vi "Max and Min (multiple).vi"(8 "error in (no error)":errorcluster, 11 "XY-data":cluster{"X-array":dbl[], "Y-array":dbl[]}[](array[cluster]) {"Y-array" format="%.2p"; "X-array" format="%.2p"}) -> (0 "error out":errorcluster, 1 "y_min (x,y)":cluster{"x":dbl, "y":dbl}[](array[cluster]), 2 "y_max (x,y)":cluster{"x":dbl, "y":dbl}[](array[cluster]), 3 "XY-data out":cluster{"X-array":dbl[], "Y-array":dbl[]}[](array[cluster]) {"Y-array" format="%.2p"; "X-array" format="%.2p"})   [LabVIEW 2019, in "xy_utilities.lvlib"]
doc: "Returns (x,y) coordinates of <b>y_max</b> and <b>y_min</b>.\n\nWire data to the data input to determine the polymorphic instance to use or manually select the instance."
uses:
  xy_utilities.lvlib
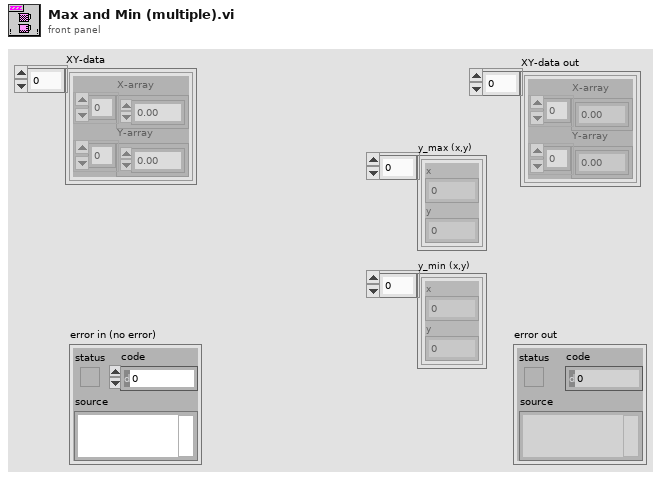
[diagram p1: front panel]
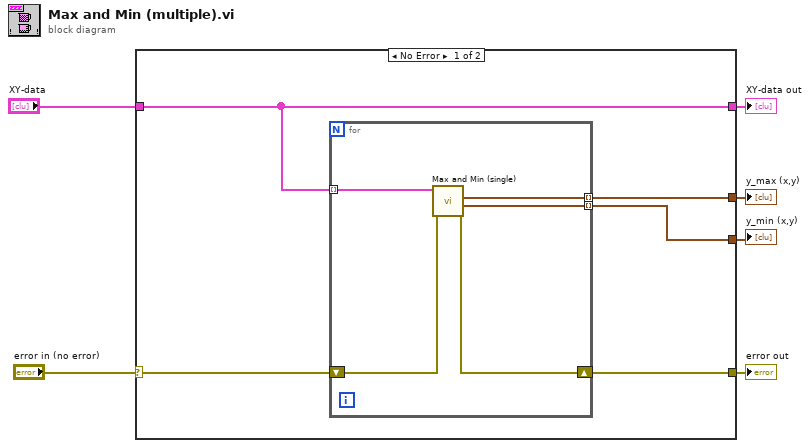
[diagram p0: block diagram]
diagram:
  n1 = case shown="No Error" "error in (no error)" {
    selector: "error in (no error)" -> [w10 w18]
    tunnel: [w9 w18] -> w5
    tunnel: "XY-data" -> [w11 w17]
    tunnel: [w11 w17] -> w3
    tunnel: [w8 _] -> w2
    tunnel: [w7 _] -> w1
    frame No Error {
      n2 = for {
        tunnel: w11 -> [w16] mode=indexing
        tunnel: [w13] -> w7 mode=indexing
        tunnel: [w12] -> w8 mode=indexing
        shift-right: [w14] -> w9
        shift-left: w10 -> [w15]
        n3 = call "Max and Min (single).vi"("error in (no error)"=w15, "XY-data"=w16) -> ("error out"=w14:errorcluster, "y_min (x,y)"=w13:cluster{"x":dbl, "y":dbl}, "y_max (x,y)"=w12:cluster{"x":dbl, "y":dbl})  [unwired: 6 in, 1 out]
      }
    }
    frame Error {
    }
  }
  "error out" <- w5
  "XY-data out" <- w3
  "y_max (x,y)" <- w2
  "y_min (x,y)" <- w1
